vi "SigProc_subVI scriptVariableFinder.vi"(5 "VarName":string, 8 "Variables":cluster{"VarName":string, "Var":dbl}[](array[cluster])) -> (0 "Found":bool, 2 "Var":dbl)   [LabVIEW 2018, in "Sig2MS.lvclass"]
uses:
  Sig2MS.lvclass
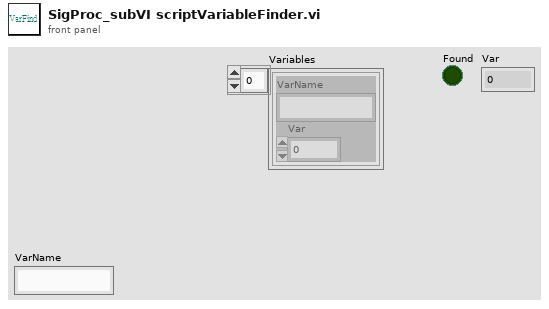
[diagram p1: front panel]
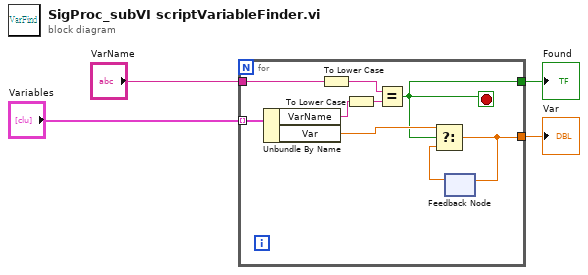
[diagram p0: block diagram]
diagram:
  n1 = for {
    tunnel: "VarName" -> [w11]
    tunnel: "Variables" -> [w13] mode=indexing
    tunnel: [w8] -> w1
    tunnel: [w7] -> w2
    stop <- w7 stop-if-true
    n2 = Unbundle By Name(w13) -> ("VarName"=w12:string, "Var"=w10:dbl)
    n3 = To Lower Case(string=w11) -> (all lower case string=w5:string)
    n4 = To Lower Case(string=w12) -> (all lower case string=w6:string)
    n5 = Equal?(x=w5, y=w6) -> (x = y?=w7:bool)
    n6 = feedback #1() -> (w9:dbl)  [unwired: 1 in]
    n7 = Select(t=w10, s=w7, f=w9) -> (s? t:f=w8:dbl)
    n8 = feedback-in #1(w8) -> ()
  }
  "Found" <- w2
  "Var" <- w1
